vi "Set Sender.vi"(10 "Sender":refnum<class "Sender.lvclass">, 11 "Has Destroyed Msg in":refnum<class "Has Destroyed Msg.lvclass">) -> (3 "Has Destroyed Msg out":refnum<class "Has Destroyed Msg.lvclass">)   [LabVIEW 2020, in "jettl.lvlib" / "Has Destroyed Msg.lvlib" / "Has Destroyed Msg.lvclass"]
uses:
  Has Destroyed Msg.lvclass
  Sender/Sender/Sender.lvclass
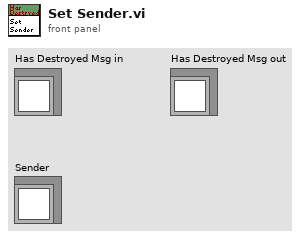
[diagram p1: front panel]
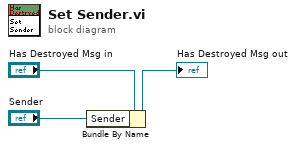
[diagram p0: block diagram]
diagram:
  n1 = Bundle By Name(cluster="Has Destroyed Msg in", "Sender"="Sender") -> (→"Has Destroyed Msg out":refnum<class "Has Destroyed Msg.lvclass">)
